vi "niRFSG Initialize.vi"(0 "resource name":refnum<k15>="pxi1slot2", 7 "id query":bool=TRUE, 9 "reset device":bool, 11 "error in":errorcluster {"code" format="%.0x"}) -> (4 "instrument handle":refnum<k15>, 15 "error out":errorcluster {"code" format="%.0x"})   [LabVIEW 2014]
doc: "Opens a session to the device you specify as the <B>resource name</B> and returns an <B>instrument handle</B> that you use to identify the NI-RFSG device in all subsequent NI-RFSG VIs.\n\n<B>Supported Devices</B>: NI 5610/5611, NI 5644R/5645R/5646R, NI 5650/5651/5652/5654/5654 with NI 5696, NI 5670/5671/5672/5673/5673E, NI 5840"
uses:
  niRFSG.dll
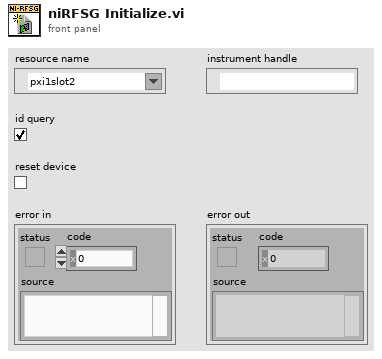
[diagram p1: front panel]
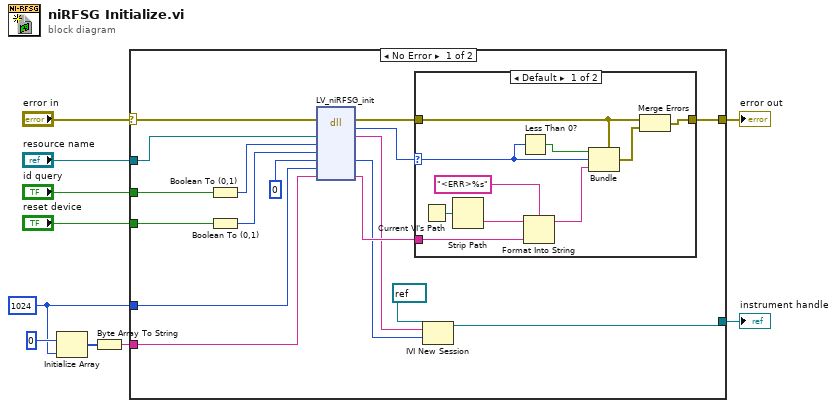
[diagram p0: block diagram]
diagram:
  w8 = 1024
  n1 = Initialize Array(u8 0, w8) -> (w10:u8[])
  n2 = Byte Array To String(unsigned byte array=w10) -> (string=w7:string)
  n3 = case shown="No Error" "error in" {
    selector: "error in" -> [w21 w39]
    tunnel: [w25 _] -> w1
    tunnel: [w22 w39] -> w2
    tunnel: "resource name" -> [w19 _]
    tunnel: "id query" -> [w24 _]
    tunnel: "reset device" -> [w23 _]
    tunnel: w8 -> [w15 _]
    tunnel: w7 -> [w14 _]
    frame No Error {
      n4 = Boolean To (0,1)(Boolean=w24) -> (0, 1=w18:i16)
      n5 = Boolean To (0,1)(Boolean=w23) -> (0, 1=w17:i16)
      n6 = dll-call lib="niRFSG**.*" fn="LV_niRFSG_init"(error in=w21, "resource name"=w19, "ID query"=w18, "reset"=w17, "instrument handle"=u32 0, "error buffer size"=w15, "error buffer"=w14) -> (error out=w20:errorcluster, "status"=w13:i32, "resource name"=w12:string, "instrument handle"=w11:u32, "error buffer"=w27:string)  [unwired: 5 in, 1 out]
      n7 = case shown="Default" w13 {
        selector: w13 -> [w31 _]
        tunnel: w27 -> [w37 _]
        tunnel: w20 -> [w29 w38]
        tunnel: [w28 w38] -> w22
        frame Default {
          n8 = Current VI's Path() -> (path=w35:path)
          n9 = Strip Path(path=w35) -> (name=w34:string)  [unwired: 1 out]
          n10 = Less Than 0?(x=w31) -> (x < 0?=w32:bool)
          n11 = Format Into String(format string="<ERR>%s", initial string=w34, w37) -> (resulting string=w33:string)  [unwired: 1 in, 1 out]
          n12 = Bundle(cluster=w29, "status"=w32, "code"=w31, "source"=w33) -> (w30:errorcluster)
          n13 = Merge Errors(w29, w30) -> (w28:errorcluster)
        }
        frame 0 {
        }
      }
      n14 = IVI New Session(9:w11, 10:w12, 11:refnum<k15> refnum ("instrument handle")) -> (3:w25:refnum<k15>)
    }
    frame Error {
    }
  }
  "instrument handle" <- w1
  "error out" <- w2
